vi "TimeTriggerToMove.vi"(9 "搬移延遲(分)":i32, 11 "Current Time":timestamp) -> (0 "目標資料夾":string, 1 "[搬移]時間點":timestamp)   [LabVIEW 2019]
panel:
  out "當前時間前十分鐘":timestamp
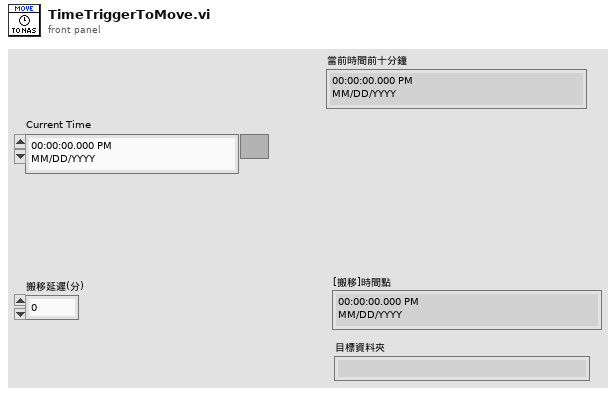
[diagram p1: front panel]
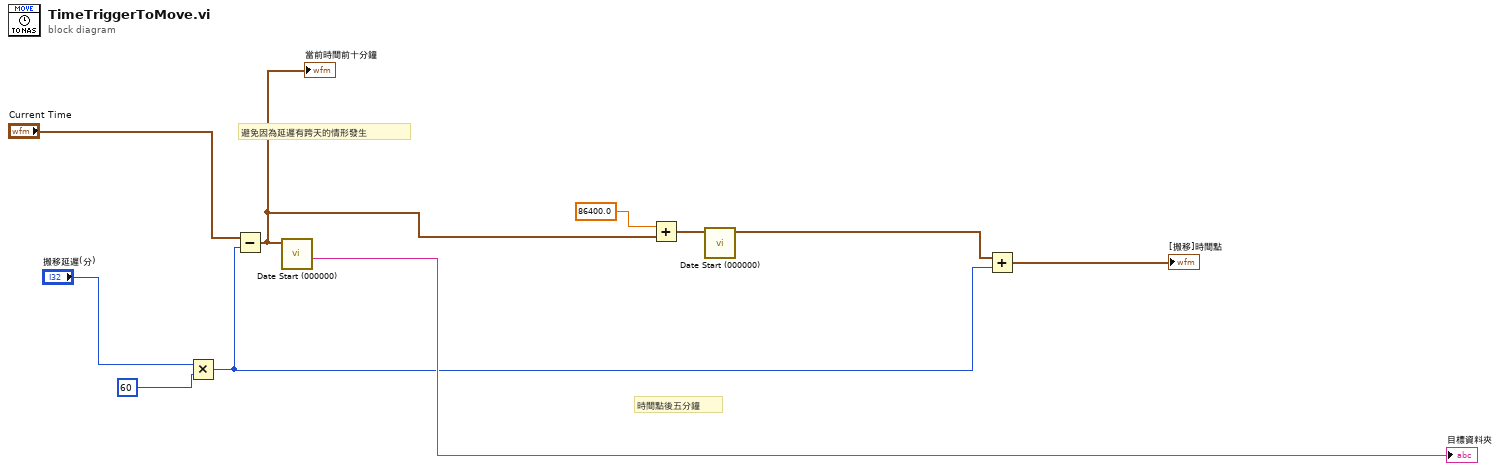
[diagram p0: block diagram]
diagram:
  # "避免因為延遲有跨天的情形發生"
  # "時間點後五分鐘"
  n1 = Multiply(x="搬移延遲(分)", y=60) -> (x*y=w2:i32)
  n2 = Subtract(x="Current Time", y=w2) -> (x-y=w3:timestamp)
  "當前時間前十分鐘" <- w3
  n3 = call "Date Start (000000).vi"("Datetime"=w3) -> ("檔名"=→"目標資料夾":string)  [unwired: 9 in, 1 out]
  n4 = Add(x=86400.0, y=w3) -> (x+y=w5:timestamp)
  n5 = call "Date Start (000000).vi"("Datetime"=w5) -> ("Date + 00:00:00"=w4:timestamp)  [unwired: 9 in, 1 out]
  n6 = Add(x=w4, y=w2) -> (x+y=→"[搬移]時間點":timestamp)
